vi "Find_Image_By_Annotation_File.vi"(6 "Array":string[](array[string]), 9 "All Files in Dir":path[](array[path]), 10 "Image/Anno Name":string, 11 "Image Path (Destination)":path) -> (1 "Anno/Img Found?":bool, 2 "Dest path":path, 3 "Source Path":path)   [LabVIEW 2020]
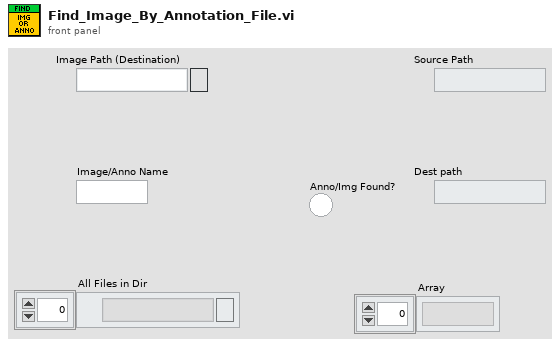
[diagram p1: front panel]
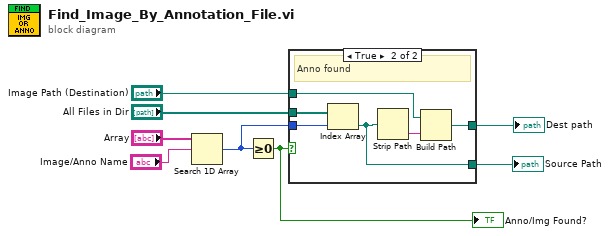
[diagram p0: block diagram]
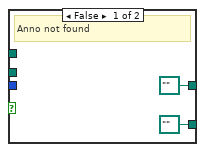
[diagram p2: hidden frame]
diagram:
  n1 = Search 1D Array(1D array="Array", element="Image/Anno Name") -> (index of element=w2:i32)  [unwired: 1 in]
  n2 = Greater Or Equal To 0?(x=w2) -> (x >= 0?=w1:bool)
  "Anno/Img Found?" <- w1
  n3 = case shown="True" w1 {
    tunnel: [path "" ("appended path") w16] -> w7
    tunnel: [path "" ("File Path") w15] -> w6
    tunnel: "All Files in Dir" -> [_ w14]
    tunnel: "Image Path (Destination)" -> [_ w13]
    tunnel: w2 -> [_ w11]
    frame False {
      # "Anno not found"
    }
    frame True {
      # "Anno found"
      n4 = Index Array(array=w14, index=w11) -> (element=w15:path)
      n5 = Strip Path(path=w15) -> (name=w12:string)  [unwired: 1 out]
      n6 = Build Path(base path=w13, name or relative path=w12) -> (appended path=w16:path)
    }
  }
  "Dest path" <- w7
  "Source Path" <- w6
